vi "Handle Error.vi"(8 "error in (no error)":errorcluster, 11 "App in":refnum<class "App.lvclass">) -> (0 "error out":errorcluster, 2 "stop actor?":bool=TRUE, 3 "App out":refnum<class "App.lvclass">)   [LabVIEW 2016, in "App.lvlib" / "App.lvclass"]
doc: "(<B>Filename</B>: Actor Framework.lvlib:Actor.lvclass:Handle Error.vi)\n\nDefines how the actor handles an error that occurred while processing a message. By default, this method does nothing except stop the actor."
uses:
  App.lvclass
  <vilib>/ActorFramework/Actor/Actor.lvclass
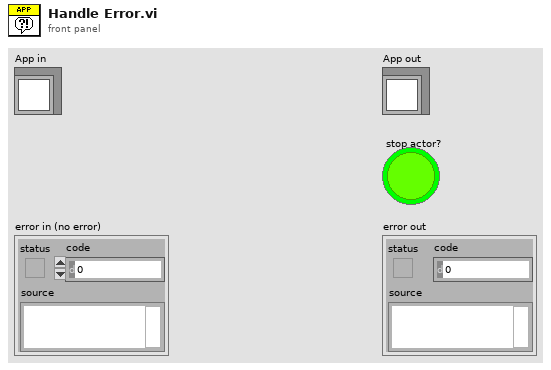
[diagram p1: front panel]
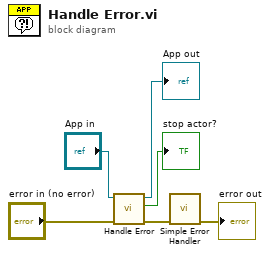
[diagram p0: block diagram]
diagram:
  n1 = call-parent "Handle Error.vi"("error in (no error)"="error in (no error)", "Actor in"="App in") -> ("error out"=w6:errorcluster, "stop actor?"=→"stop actor?":bool, "Actor out"=→"App out":refnum<class "App.lvclass">)  [unwired: 7 in]
  n2 = call <vilib>:"Simple Error Handler.vi"("error in (no error)"=w6) -> ("error out"=→"error out":errorcluster)  [unwired: 4 in, 4 out]
